vi "BATTERY EMULATOR AUTO MODE.vi"(8 "error IN":errorcluster) -> (0 "error out":errorcluster)   [LabVIEW 2018]
uses:
  Controls/MODEL CONTROL.ctl
  3e16ebac-11a9-43af-ac05-86c9ef550ade.vi
  17a302df-ff61-441d-8d7b-7ff2f5324251.vi
  a2baa657-6743-459a-891e-8081dcc02569.vi
  93341af7-0d01-4cec-89d3-509ad52480dd.vi
  <vilib>/xnet/xnet.llb/XNET Create Session (Signal Input Single-point).vi
  <vilib>/xnet/xnet.llb/XNET Read (Signal Single-point).vi
  <vilib>/xnet/xnet.llb/XNET Create Session (Signal Output Single-point).vi
  <vilib>/xnet/xnet.llb/XNET Write (Signal Single-point).vi
panel:
  in  "UPLOAD DATA":bool
  out "MESSAGES":string
  out "CP POWER":string
  out "CP CURRENT":string
  out "CP VOLTAGE":string
  out "CI POWER":string
  out "CI CURRENT":string
  out "CI VOLTAGE":string
  out "CV POWER":string
  out "CV CURRENT":string
  out "CV VOLTAGE":string
  out "CONTROL SELECTION":string
  out "HVHC SELECTION":string
  in  "CP POWER":string
  in  "CP CURRENT":string
  in  "CP VOLTAGE":string
  in  "CI POWER":string
  in  "CI CURRENT":string
  in  "CI VOLTAGE":string
  in  "CV POWER":string
  in  "CV CURRENT":string
  in  "CV VOLTAGE":string
  in  "CONTROL SELECTION":string(combo)
  in  "HVHC SELECTION":string(combo)
  out "Headline":string
  in  "Save Button":bool
  in  "MODEL SELECTION":string(combo)
  # "BATTERY EMULATOR CONTROLS"
  # "BATTERY EMULATOR DATA"
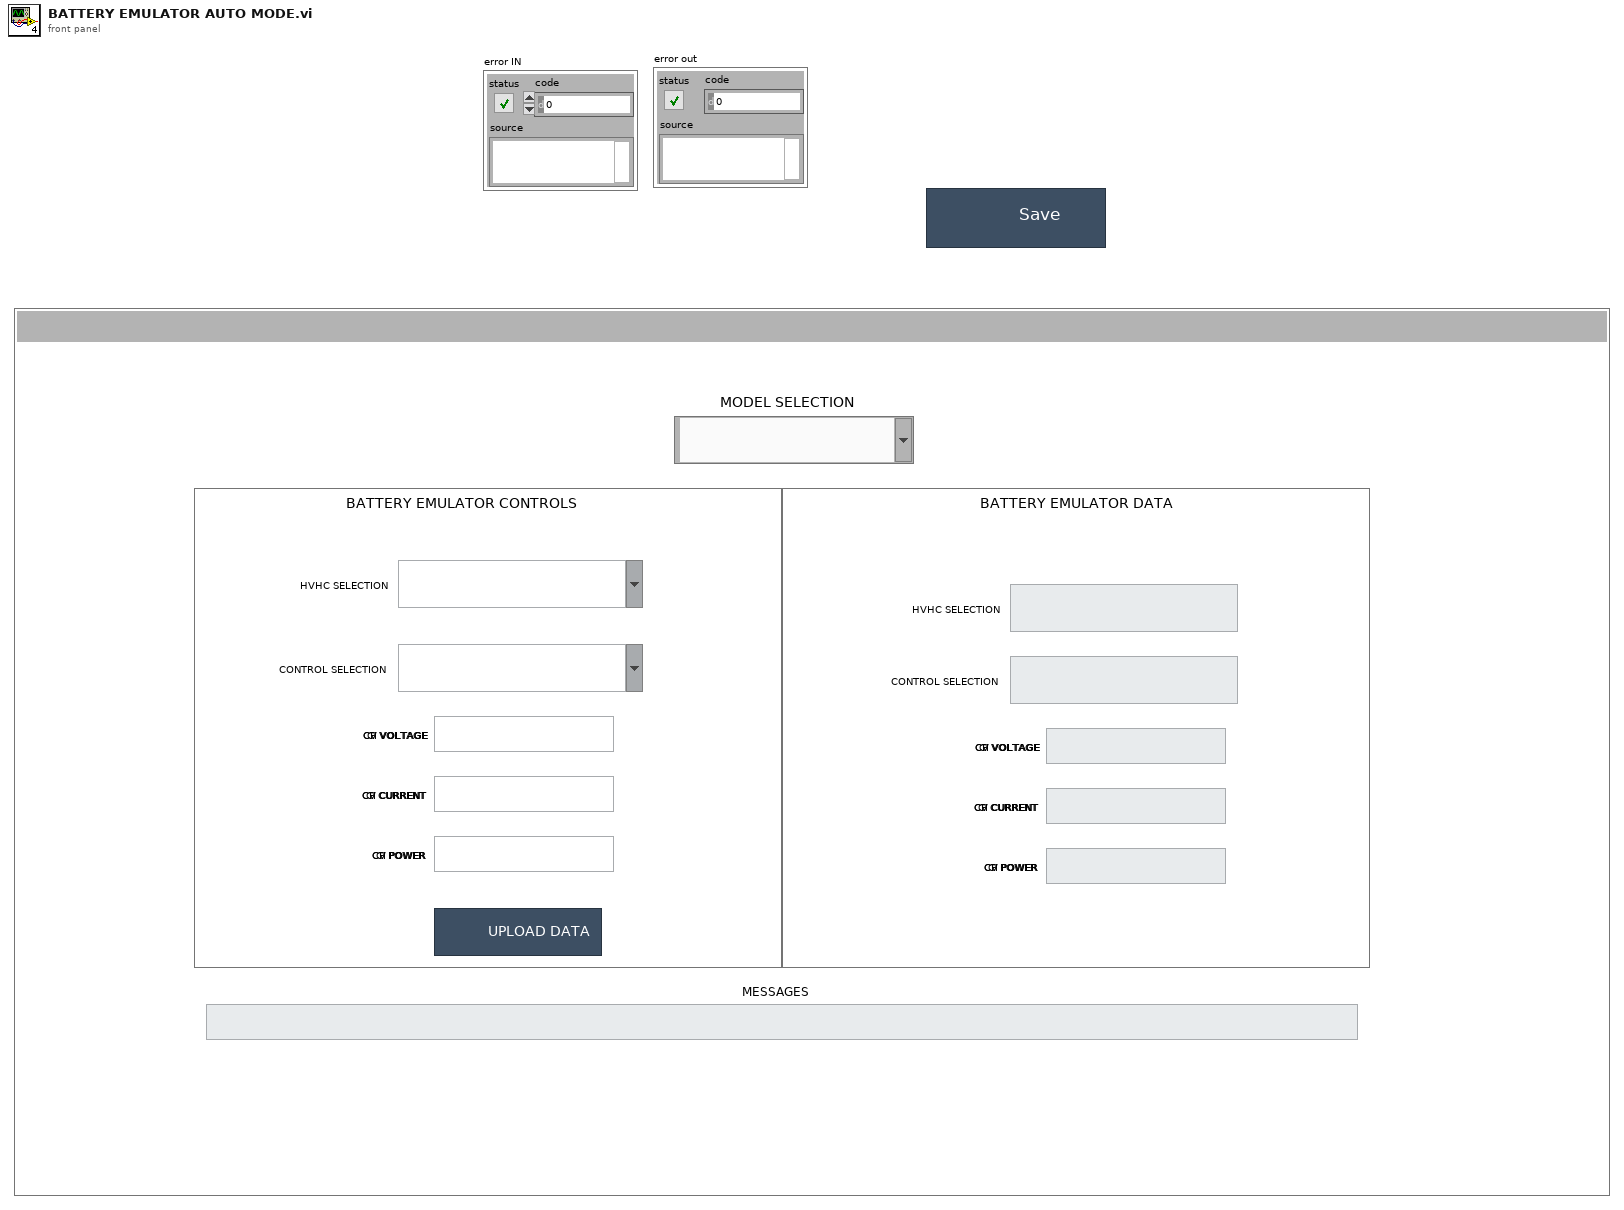
[diagram p1: front panel]
types:
  T1 = enum32{"Invalid", "Standard", "Closed", "Hidden", "Minimized", "Maximized"}
  T2 = enum32{"invalid app kind", "Development System", "Run Time System", "Student Edition", "Embedded LabVIEW", "Evaluation", "Custom"}
  T3 = typedef "MODEL CONTROL.ctl" = enum16{"OPEN", "READ", "WRITE", "CLOSE"}
  T4 = cluster{"Core":cluster{"Current VI Reference":refnum<vi>, "Close Panel on Exit?":bool}, "CHANGE REQ?":bool, "Your string data":string, "BATTERY EMULATOR":cluster{"HVHC SELECT":string, "CONTROL SELECTION":string, "CV VOLTAGE":string, "CV CURRENT":string, "CV POWER":string, "CI VOLTAGE":string, "CI CURRENT":string, "CI POWER":string, "CP VOLTAGE":string, "CP CURRENT":string, "CP POWER":string}, "File paths":cluster{"Base file path":path, "Model File path":path}, "DATA WRITE COUNT":i32, "MESSAGES":string}
  T5 = cluster{"HVHC SELECT":string, "CONTROL SELECTION":string, "CV VOLTAGE":string, "CV CURRENT":string, "CV POWER":string, "CI VOLTAGE":string, "CI CURRENT":string, "CI POWER":string, "CP VOLTAGE":string, "CP CURRENT":string, "CP POWER":string}
  T6 = cluster{"Base file path":path, "Model File path":path}
  T7 = cluster{"Current VI Reference":refnum<vi>, "Close Panel on Exit?":bool}
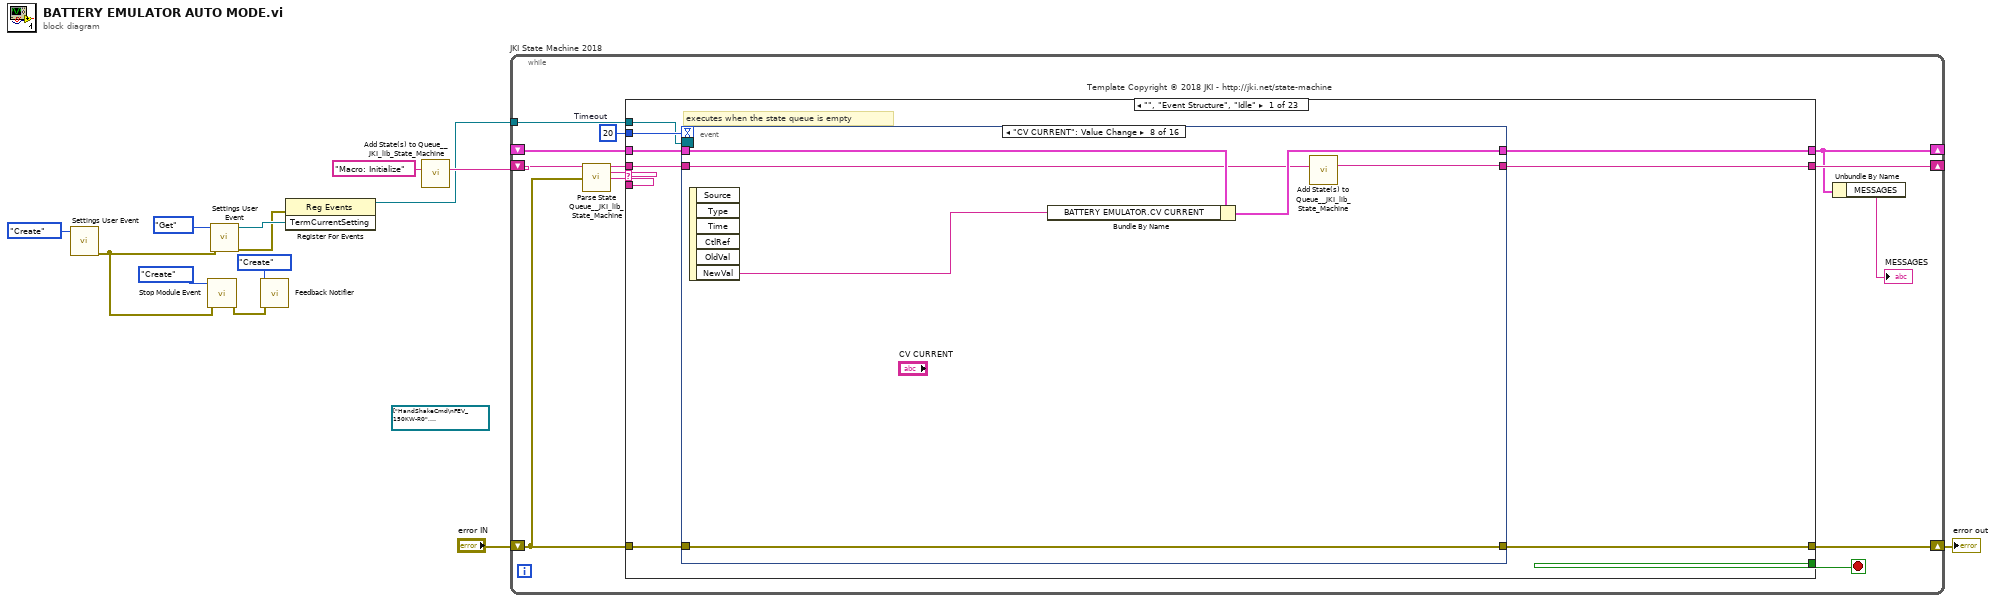
[diagram p0: block diagram]
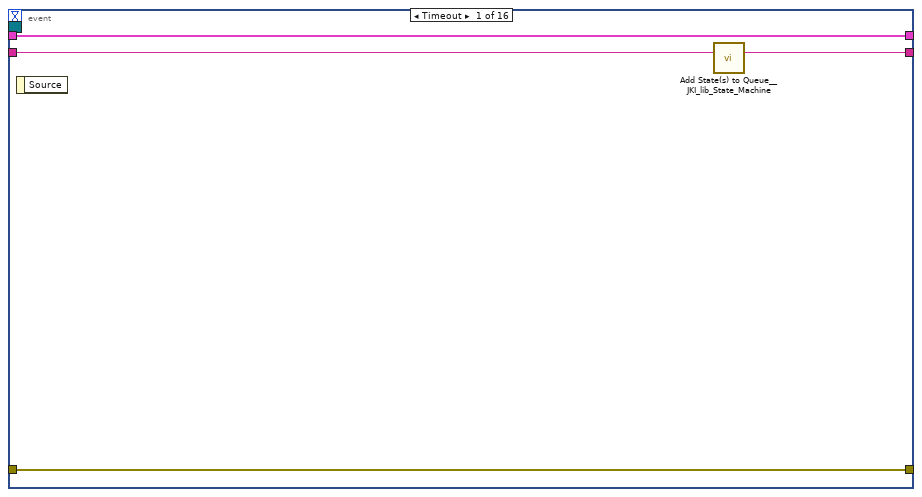
[diagram p2: hidden frame]
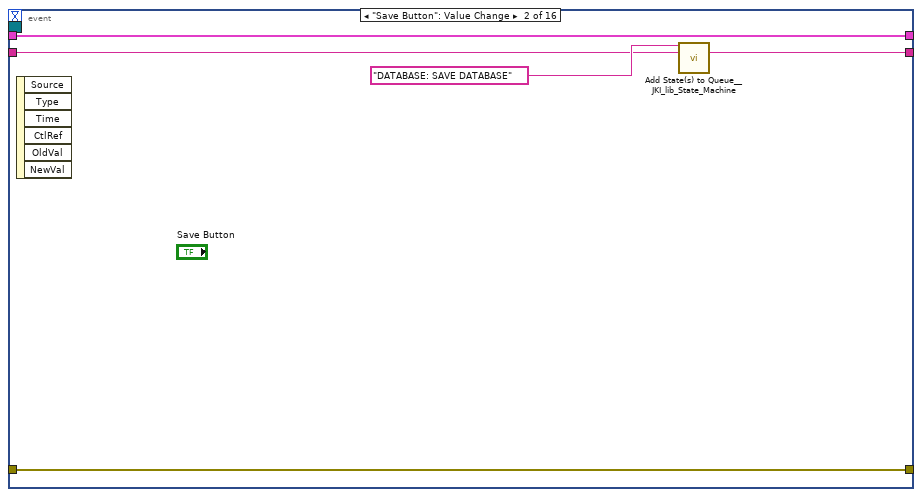
[diagram p3: hidden frame]
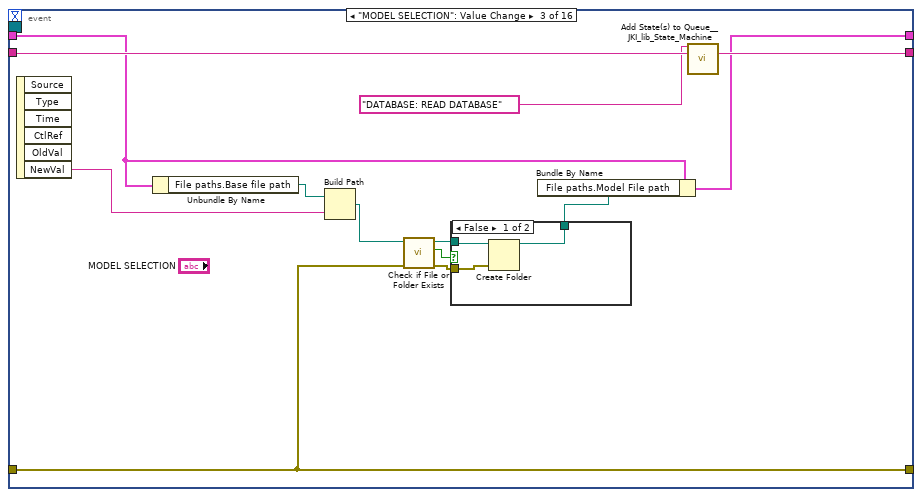
[diagram p4: hidden frame]
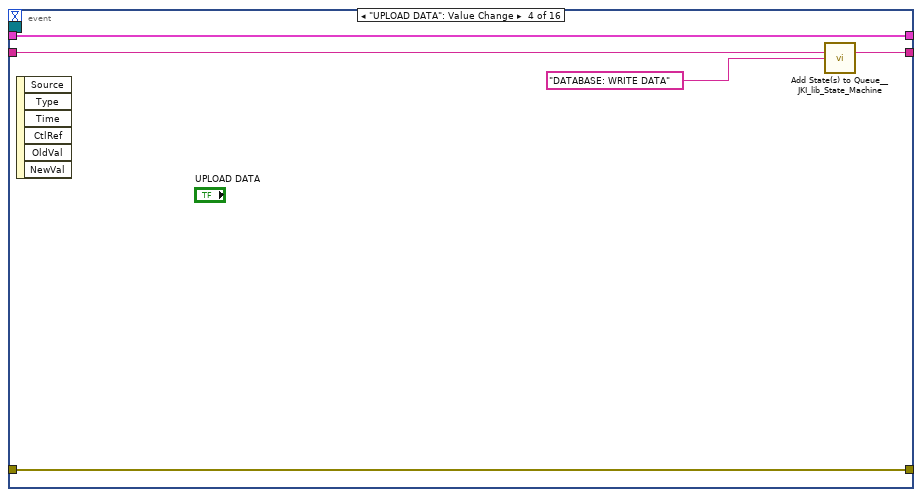
[diagram p6: hidden frame]
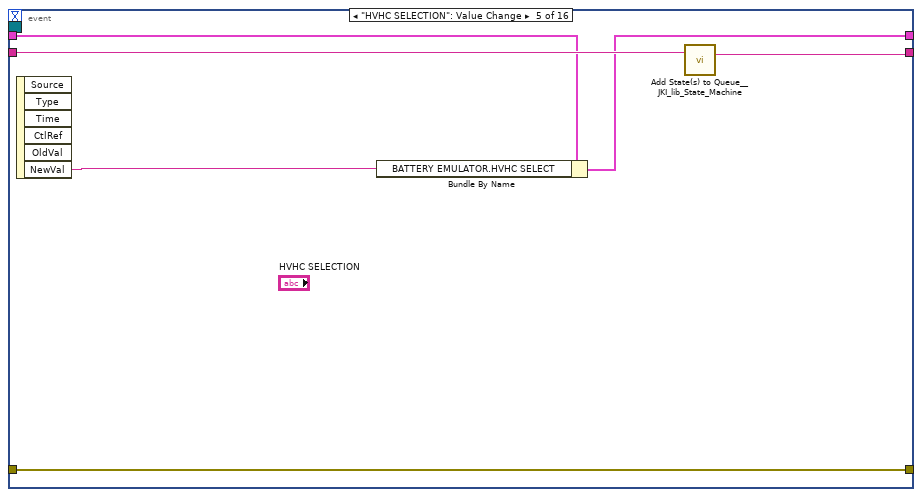
[diagram p7: hidden frame]
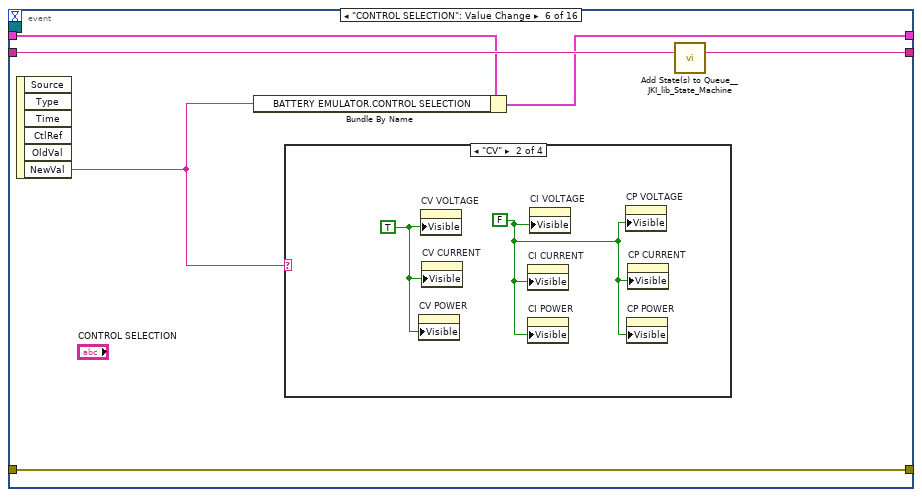
[diagram p8: hidden frame]
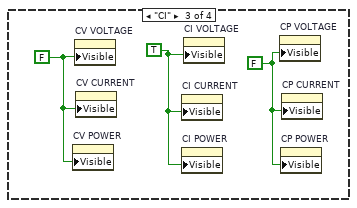
[diagram p10: hidden frame]
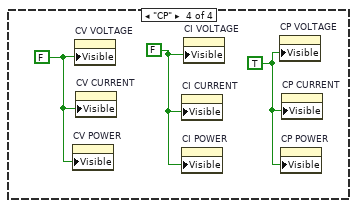
[diagram p11: hidden frame]
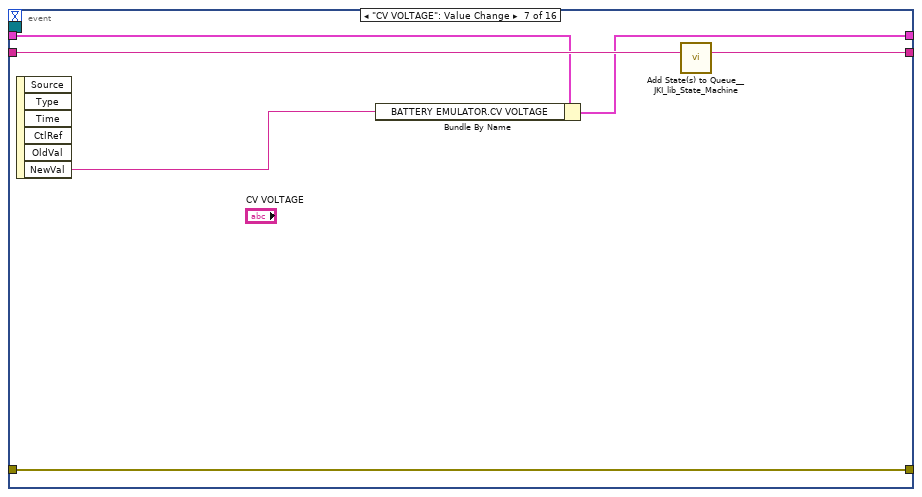
[diagram p12: hidden frame]
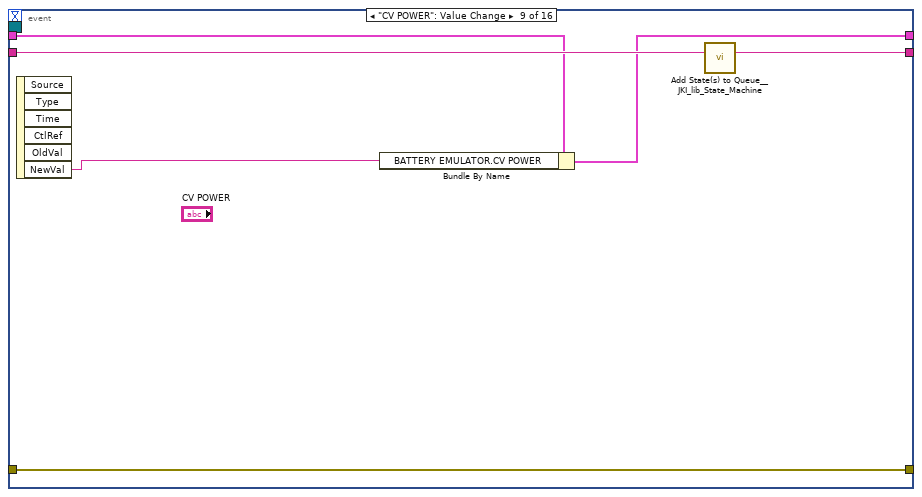
[diagram p13: hidden frame]
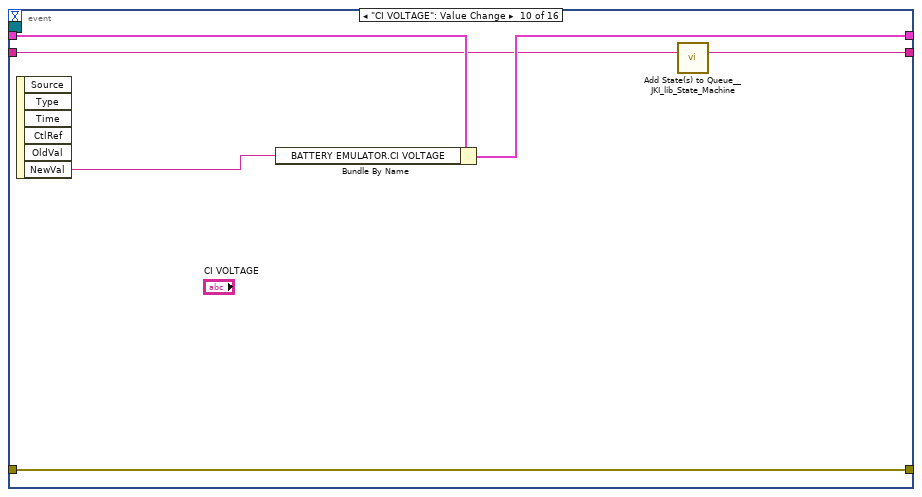
[diagram p14: hidden frame]
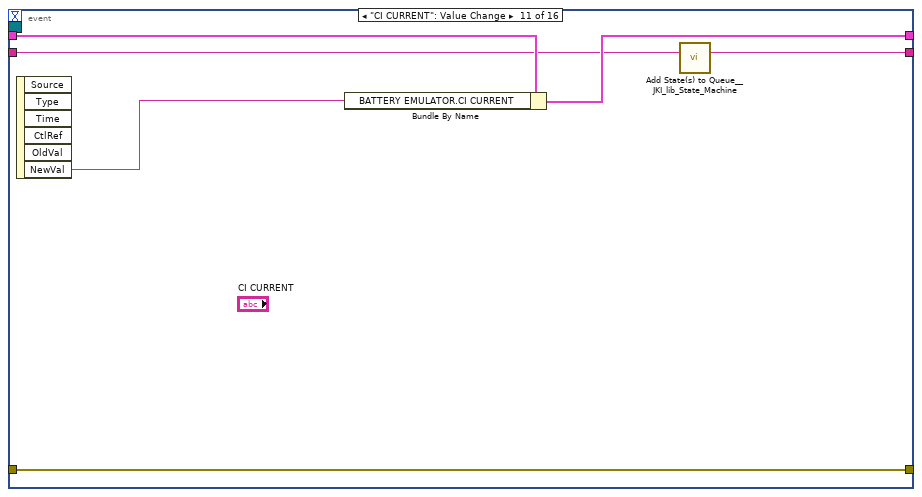
[diagram p15: hidden frame]
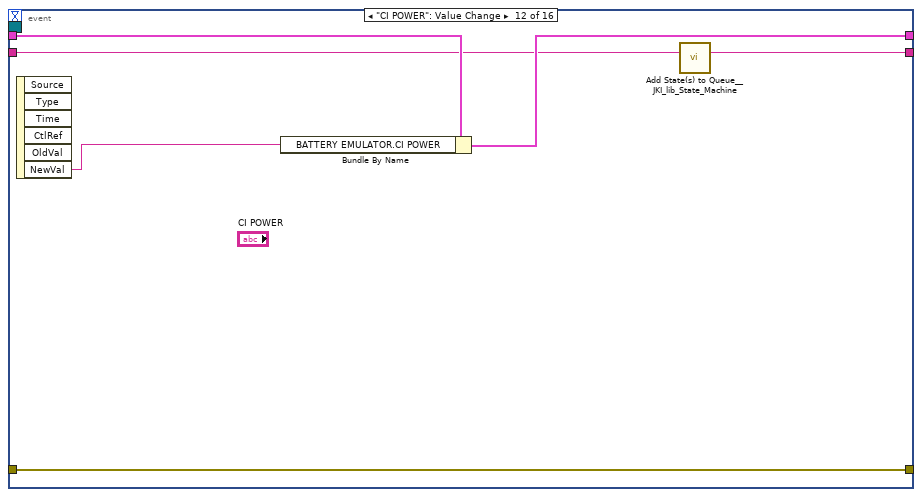
[diagram p16: hidden frame]
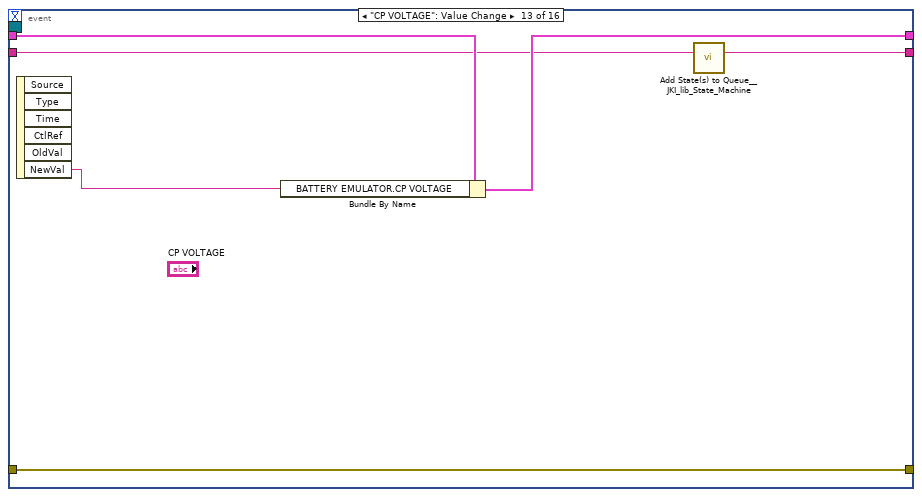
[diagram p17: hidden frame]
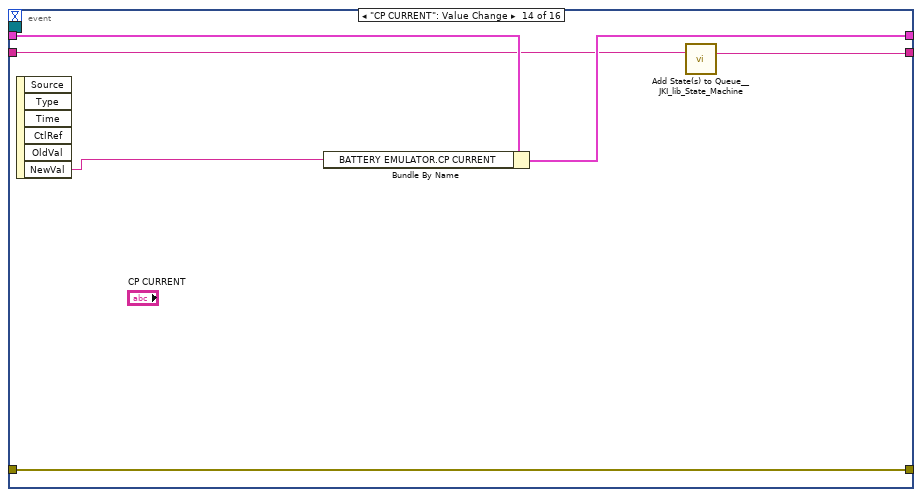
[diagram p18: hidden frame]
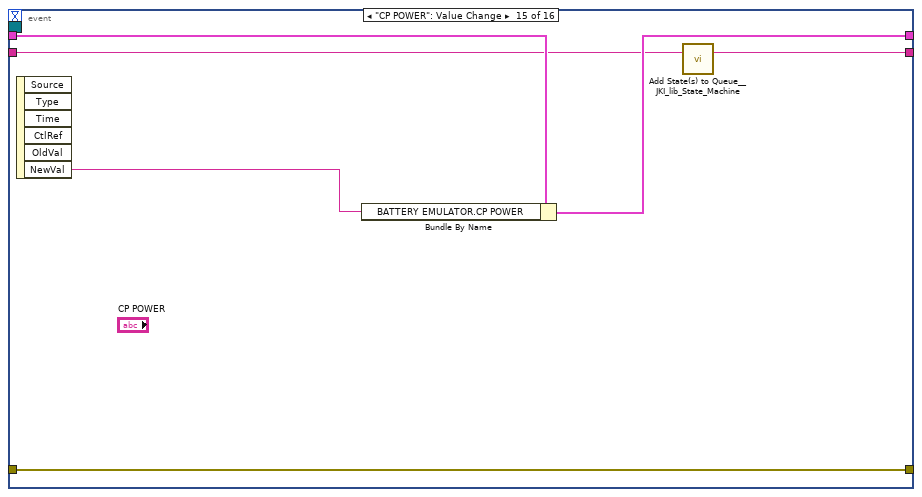
[diagram p19: hidden frame]
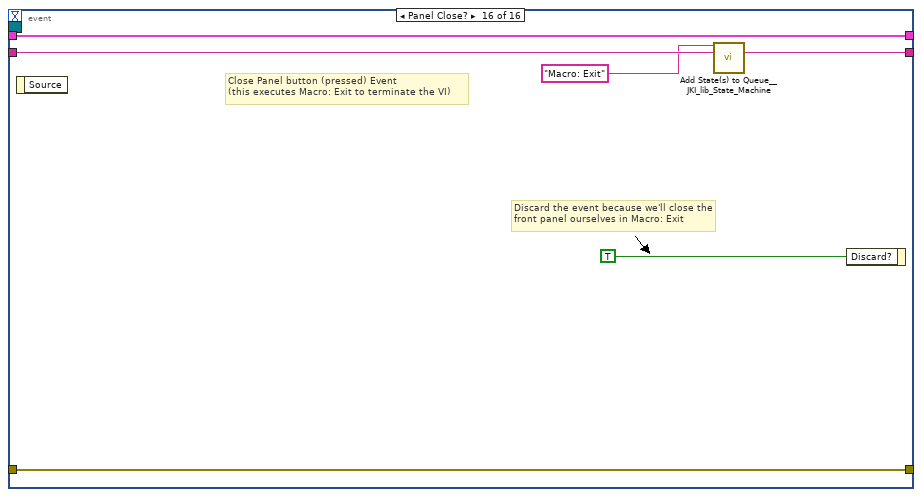
[diagram p20: hidden frame]
diagram:
  (unwired) refnum<k21>[] ["HandShakeCmd\nFEV_150KW-R0", "RemoteDisplaySel\nFEV_150KW-R0", "Select_HVHC", "Select_CVCICP", "CV_SetCurrentLimit\nFEV_150KW-R0", "CV_SetPowerLimit\nFEV_150KW-R0", "CV_SetVoltage\nFEV_150KW-R0", "B_RemoteToDcps.Reserved\nFEV_150KW-R0", "CI_SetCurrent\nFEV_150KW-R0", "CI_SetPowerLimit\nFEV_150KW-R0", "CI_SetVoltageLimit\nFEV_150KW-R0", "C_RemoteToDcps.Reserved\nFEV_150KW-R0", "CP_SetCurrentLimit\nFEV_150KW-R0", "CP_SetPower\nFEV_150KW-R0", "CP_SetVoltageLimit\nFEV_150KW-R0", "D_RemoteToDcps.UpdateCmd\nFEV_150KW-R0", "HandShakeAcknowledge\nFEV_150KW-R0", "RemoteDisplaySelAck\nFEV_150KW-R0", "Select_CVCICPAck\nFEV_150KW-R0", "Select_HVHC_Ack\nFEV_150KW-R0", "CV_SetCurrentLimitAck\nFEV_150KW-R0", "CV_SetPowerLimitAck\nFEV_150KW-R0", "CV_SetVoltageAck\nFEV_150KW-R0", "PowerSwitchONStatus\nFEV_150KW-R0", "CI_SetCurrentAck\nFEV_150KW-R0", "CI_SetPowerLimitAck\nFEV_150KW-R0", "CI_SetVoltageLimitAck\nFEV_150KW-R0", "ErrorControlSelErr\nFEV_150KW-R0", "ErrorCurSetOutofRange\nFEV_150KW-R0", "ErrorNotInRemoteMode\nFEV_150KW-R0", "ErrorPowerSetOutofRange\nFEV_150KW-R0", "ErrorVoltSetOutofRange\nFEV_150KW-R0", "ErrorWrongHVSel\nFEV_150KW-R0", "Reserved_Status\nFEV_150KW-R0", "CP_SetCurrentLimitAck\nFEV_150KW-R0", "CP_SetPowerAck\nFEV_150KW-R0", "CP_SetVoltageLimitAck\nFEV_150KW-R0", "UpdateCmdAcknowledge\nFEV_150KW-R0", "OutputCurrent\nFEV_150KW-R0", "OutputPower\nFEV_150KW-R0", "OutputVoltage\nFEV_150KW-R0", "StatusDcpsFault\nFEV_150KW-R0", "StatusDcpsON\nFEV_150KW-R0", "StatusDcpsOverload\nFEV_150KW-R0", "StatusDcpsTrip\nFEV_150KW-R0", "StatusHCHV_selection\nFEV_150KW-R0", "StatusInputOverVolt\nFEV_150KW-R0", "StatusInputUnderVolt\nFEV_150KW-R0", "StatusMainsHealthy\nFEV_150KW-R0", "StatusOutputOverVolt\nFEV_150KW-R0", "StatusOutputUnderVolt\nFEV_150KW-R0", "StatusOverTemperature\nFEV_150KW-R0", "StatusRemoteLocal\nFEV_150KW-R0"] ("Sigs 3")
  n1 = call "Settings User Event.vi"("Action"=enum16{"Create", "Get", "Destroy"}."Create") -> ("error out"=w6:errorcluster)  [unwired: 9 in, 1 out]
  n2 = call "Stop Module Event.vi"("error in (no error)"=w6, "Action"=enum16{"Create", "Get", "Destroy"}."Create") -> ("error out"=w5:errorcluster)  [unwired: 8 in, 1 out]
  n3 = call "Settings User Event.vi"("error in (no error)"=w6, "Action"=enum16{"Create", "Get", "Destroy"}."Get") -> ("error out"=w8:errorcluster, "TermCurrentSetting"=w9:refnum<user-event>)  [unwired: 8 in]
  n4 = call "Feedback Notifier.vi"("error in (no error)"=w5, "Action"=enum16{"Create", "Get", "Destroy"}."Create") -> ()  [unwired: 8 in, 2 out]
  n5 = register-events(error in=w8, w9) -> (reference out=w3:refnum<event-registration>)  [unwired: 1 in, 1 out]
  n6 = call <vilib>:"Add State(s) to Queue__JKI_lib_State_Machine.vi"("State(s) in (\"\")"="Macro: Initialize") -> ("States Out"=w13:string)  [unwired: 14 in]
  n7 = while "JKI State Machine 2018" {
    shift-right: [w15] -> _
    shift-left: _ -> [w19]
    shift-right: [w22] -> w1
    shift-left: "error IN" -> [w17]
    shift-right: [w21] -> _
    shift-left: w13 -> [w23]
    tunnel: w3 -> [w16]
    stop <- w20 stop-if-true
    w18 = 20  # Timeout
    # "Template Copyright © 2018 JKI - http://jki.net/state-machine"
    n8 = call <vilib>:"Parse State Queue__JKI_lib_State_Machine.vi"("State Queue"=w23, "Error In (no error)"=w17) -> ("Remaining States"=w25:string, "Current State"=w26:string, "Arguments"=w24:string)  [unwired: 11 in]
    n9 = case shown="\"\", \"Event Structure\", \"Idle\"" w26 {
      selector: w26 -> [_ _ w150 _ _ _ _ _ _ _ _ _ _ _ _ _ _ _ _ _ _ _ _]
      tunnel: w25 -> [w34 w149 w154 w173 w179 w184 w188 w199 w205 w209 w213 w219 w223 w226 w249 w261 w330 w335 w352 w366 w391 w438 w506]
      tunnel: w24 -> [_ _ _ _ _ _ _ _ _ _ _ _ _ _ w244 w255 _ _ _ _ _ _ _]
      tunnel: w19 -> [w32 w146 w152 w166 w176 w182 w185 _ w200 w206 w211 w217 w220 w238 w247 w257 w327 w332 w340 w363 w370 w402 w476]
      tunnel: [w31 w147 w156 w170 errorcluster {"status"=FALSE, "code"=0, "source"=""} ("error out") w181 w186 w196 w201 w207 w210 w214 w221 w239 w245 w258 w328 w333 w344 w364 w385 w428 w477] -> w22
      tunnel: w17 -> [w30 w147 w155 w170 w175 w181 w186 w196 w202 w207 w210 w215 w221 w236 w246 w259 w328 w333 w345 w364 w389 w410 w478]
      tunnel: [w33 w148 w153 w172 w178 w183 w187 w198 w204 w208 w212 w218 w222 w243 w248 w260 w329 w334 w351 w365 w390 w437 w505] -> w21
      tunnel: [_ _ _ _ _ TRUE _ _ _ _ _ _ _ _ _ _ _ _ _ _ _ _ _] -> w20
      tunnel: [w29 w146 w152 w171 w176 w182 w185 w197 w200 w206 w211 w217 w220 w237 w247 w257 w327 w332 w339 w363 w369 w401 w476] -> w15
      tunnel: w18 -> [w28 _ _ _ _ _ _ _ _ _ _ _ _ _ _ _ _ _ _ _ _ _ _]
      tunnel: w16 -> [w27 _ _ _ _ _ _ _ _ _ _ w216 _ _ _ _ _ _ _ _ _ _ _]
      frame "", "Event Structure", "Idle" {
        # "executes when the state queue is empty"
        n10 = event shown="[7] \"CV CURRENT\": Value Change" {
          selector: w27 -> [_ _ _ _ _ _ _ _ _ _ _ _ _ _ _ _]
          dyn-events: _ -> [_ _ _ _ _ _ _ _ _ _ _ _ _ _ _ _]
          timeout: w28 -> [_ _ _ _ _ _ _ _ _ _ _ _ _ _ _ _]
          tunnel: w34 -> [w38 w40 w55 w63 w70 w75 w90 w93 w101 w105 w111 w116 w122 w128 w134 w145]
          tunnel: [w37 w41 w56 w64 w71 w76 w91 w94 w102 w106 w112 w117 w123 w129 w135 w144] -> w33
          tunnel: w32 -> [w35 w42 w51 w65 w69 w74 w89 w97 w100 w109 w114 w120 w126 w132 w138 w142]
          tunnel: [w36 w39 w48 w62 w66 w77 w86 w92 w103 w104 w115 w121 w127 w133 w139 w143] -> w31
          tunnel: w30 -> [w36 w39 w48 w62 w66 w77 w86 w92 w103 w104 w115 w121 w127 w133 w139 w143]
          tunnel: [w35 w42 w50 w65 w67 w73 w87 w96 w99 w108 w113 w118 w125 w131 w137 w142] -> w29
          event Timeout {
            n11 = event-data() -> ()  [unwired: 1 in, 1 out]
            n12 = call <vilib>:"Add State(s) to Queue__JKI_lib_State_Machine.vi"("State(s) in (\"\")"=w38) -> ("States Out"=w37:string)  [unwired: 14 in]
          }
          event "Save Button": Value Change {
            n13 = event-data() -> ()  [unwired: 1 in, 6 out]
            n14 = call <vilib>:"Add State(s) to Queue__JKI_lib_State_Machine.vi"("State(s) in Front (\"\")"="DATABASE: SAVE DATABASE", "State(s) in (\"\")"=w40) -> ("States Out"=w41:string)  [unwired: 13 in]
          }
          event "MODEL SELECTION": Value Change {
            n15 = event-data() -> ("NewVal"=w52:string)  [unwired: 1 in, 5 out]
            n16 = Unbundle By Name(w51) -> ("File paths.Base file path"=w53:path)
            n17 = Build Path(base path=w53, name or relative path=w52) -> (appended path=w49:path)
            n18 = call <vilib>:"Check if File or Folder Exists.vi"("error in (no error)"=w48, "path"=w49) -> ("error out"=w46:errorcluster, "file or folder exists?"=w45:bool, "dup path"=w47:path)  [unwired: 7 in]
            n19 = case shown="False" w45 {
              tunnel: w47 -> [w58 w60]
              tunnel: w46 -> [w59 _]
              tunnel: [w57 w60] -> w44
              frame False {
                n20 = Create Folder(path (use dialog)=w58, error in=w59) -> (created path=w57:path)  [unwired: 1 in, 2 out]
              }
              frame True {
              }
            }
            n21 = Bundle By Name(cluster=w51, "File paths.Model File path"=w44) -> (w50:T4)
            n22 = call <vilib>:"Add State(s) to Queue__JKI_lib_State_Machine.vi"("State(s) in Front (\"\")"="DATABASE: READ DATABASE", "State(s) in (\"\")"=w55) -> ("States Out"=w56:string)  [unwired: 13 in]
          }
          event "UPLOAD DATA": Value Change {
            n23 = event-data() -> ()  [unwired: 1 in, 6 out]
            n24 = call <vilib>:"Add State(s) to Queue__JKI_lib_State_Machine.vi"("State(s) in (\"\")"=w63, "State(s) at Back (\"\")"="DATABASE: WRITE DATA") -> ("States Out"=w64:string)  [unwired: 13 in]
          }
          event "HVHC SELECTION": Value Change {
            n25 = event-data() -> ("NewVal"=w68:string)  [unwired: 1 in, 5 out]
            n26 = Bundle By Name(cluster=w69, "BATTERY EMULATOR.HVHC SELECT"=w68) -> (w67:T4)
            n27 = call <vilib>:"Add State(s) to Queue__JKI_lib_State_Machine.vi"("State(s) in (\"\")"=w70) -> ("States Out"=w71:string)  [unwired: 14 in]
          }
          event "CONTROL SELECTION": Value Change {
            n28 = event-data() -> ("NewVal"=w72:string)  [unwired: 1 in, 5 out]
            n29 = Bundle By Name(cluster=w74, "BATTERY EMULATOR.CONTROL SELECTION"=w72) -> (w73:T4)
            n30 = case shown="\"CV\"" w72 {
              frame "False", Default {
              }
              frame "CV" {
                w78 = FALSE ("Visible")
                w79 = TRUE ("Visible")
                n31 = property on="CV POWER" class="Str"("Visible"=w79) -> ()  [unwired: 2 in, 2 out]
                n32 = property on="CV VOLTAGE" class="Str"("Visible"=w79) -> ()  [unwired: 2 in, 2 out]
                n33 = property on="CV CURRENT" class="Str"("Visible"=w79) -> ()  [unwired: 2 in, 2 out]
                n34 = property on="CI CURRENT" class="Str"("Visible"=w78) -> ()  [unwired: 2 in, 2 out]
                n35 = property on="CI POWER" class="Str"("Visible"=w78) -> ()  [unwired: 2 in, 2 out]
                n36 = property on="CI VOLTAGE" class="Str"("Visible"=w78) -> ()  [unwired: 2 in, 2 out]
                n37 = property on="CP VOLTAGE" class="Str"("Visible"=w78) -> ()  [unwired: 2 in, 2 out]
                n38 = property on="CP POWER" class="Str"("Visible"=w78) -> ()  [unwired: 2 in, 2 out]
                n39 = property on="CP CURRENT" class="Str"("Visible"=w78) -> ()  [unwired: 2 in, 2 out]
              }
              frame "CI" {
                w80 = FALSE ("Visible")
                w81 = TRUE ("Visible")
                w82 = FALSE ("Visible")
                n40 = property on="CV POWER" class="Str"("Visible"=w82) -> ()  [unwired: 2 in, 2 out]
                n41 = property on="CV VOLTAGE" class="Str"("Visible"=w82) -> ()  [unwired: 2 in, 2 out]
                n42 = property on="CV CURRENT" class="Str"("Visible"=w82) -> ()  [unwired: 2 in, 2 out]
                n43 = property on="CI CURRENT" class="Str"("Visible"=w81) -> ()  [unwired: 2 in, 2 out]
                n44 = property on="CI POWER" class="Str"("Visible"=w81) -> ()  [unwired: 2 in, 2 out]
                n45 = property on="CI VOLTAGE" class="Str"("Visible"=w81) -> ()  [unwired: 2 in, 2 out]
                n46 = property on="CP VOLTAGE" class="Str"("Visible"=w80) -> ()  [unwired: 2 in, 2 out]
                n47 = property on="CP POWER" class="Str"("Visible"=w80) -> ()  [unwired: 2 in, 2 out]
                n48 = property on="CP CURRENT" class="Str"("Visible"=w80) -> ()  [unwired: 2 in, 2 out]
              }
              frame "CP" {
                w83 = TRUE ("Visible")
                w84 = FALSE ("Visible")
                w85 = FALSE ("Visible")
                n49 = property on="CV POWER" class="Str"("Visible"=w85) -> ()  [unwired: 2 in, 2 out]
                n50 = property on="CV VOLTAGE" class="Str"("Visible"=w85) -> ()  [unwired: 2 in, 2 out]
                n51 = property on="CV CURRENT" class="Str"("Visible"=w85) -> ()  [unwired: 2 in, 2 out]
                n52 = property on="CI CURRENT" class="Str"("Visible"=w84) -> ()  [unwired: 2 in, 2 out]
                n53 = property on="CI POWER" class="Str"("Visible"=w84) -> ()  [unwired: 2 in, 2 out]
                n54 = property on="CI VOLTAGE" class="Str"("Visible"=w84) -> ()  [unwired: 2 in, 2 out]
                n55 = property on="CP VOLTAGE" class="Str"("Visible"=w83) -> ()  [unwired: 2 in, 2 out]
                n56 = property on="CP POWER" class="Str"("Visible"=w83) -> ()  [unwired: 2 in, 2 out]
                n57 = property on="CP CURRENT" class="Str"("Visible"=w83) -> ()  [unwired: 2 in, 2 out]
              }
            }
            n58 = call <vilib>:"Add State(s) to Queue__JKI_lib_State_Machine.vi"("State(s) in (\"\")"=w75) -> ("States Out"=w76:string)  [unwired: 14 in]
          }
          event "CV VOLTAGE": Value Change {
            n59 = event-data() -> ("NewVal"=w88:string)  [unwired: 1 in, 5 out]
            n60 = Bundle By Name(cluster=w89, "BATTERY EMULATOR.CV VOLTAGE"=w88) -> (w87:T4)
            n61 = call <vilib>:"Add State(s) to Queue__JKI_lib_State_Machine.vi"("State(s) in (\"\")"=w90) -> ("States Out"=w91:string)  [unwired: 14 in]
          }
          event "CV CURRENT": Value Change {
            n62 = event-data() -> ("NewVal"=w95:string)  [unwired: 1 in, 5 out]
            n63 = Bundle By Name(cluster=w97, "BATTERY EMULATOR.CV CURRENT"=w95) -> (w96:T4)
            n64 = call <vilib>:"Add State(s) to Queue__JKI_lib_State_Machine.vi"("State(s) in (\"\")"=w93) -> ("States Out"=w94:string)  [unwired: 14 in]
          }
          event "CV POWER": Value Change {
            n65 = event-data() -> ("NewVal"=w98:string)  [unwired: 1 in, 5 out]
            n66 = Bundle By Name(cluster=w100, "BATTERY EMULATOR.CV POWER"=w98) -> (w99:T4)
            n67 = call <vilib>:"Add State(s) to Queue__JKI_lib_State_Machine.vi"("State(s) in (\"\")"=w101) -> ("States Out"=w102:string)  [unwired: 14 in]
          }
          event "CI VOLTAGE": Value Change {
            n68 = event-data() -> ("NewVal"=w107:string)  [unwired: 1 in, 5 out]
            n69 = Bundle By Name(cluster=w109, "BATTERY EMULATOR.CI VOLTAGE"=w107) -> (w108:T4)
            n70 = call <vilib>:"Add State(s) to Queue__JKI_lib_State_Machine.vi"("State(s) in (\"\")"=w105) -> ("States Out"=w106:string)  [unwired: 14 in]
          }
          event "CI CURRENT": Value Change {
            n71 = event-data() -> ("NewVal"=w110:string)  [unwired: 1 in, 5 out]
            n72 = Bundle By Name(cluster=w114, "BATTERY EMULATOR.CI CURRENT"=w110) -> (w113:T4)
            n73 = call <vilib>:"Add State(s) to Queue__JKI_lib_State_Machine.vi"("State(s) in (\"\")"=w111) -> ("States Out"=w112:string)  [unwired: 14 in]
          }
          event "CI POWER": Value Change {
            n74 = event-data() -> ("NewVal"=w119:string)  [unwired: 1 in, 5 out]
            n75 = Bundle By Name(cluster=w120, "BATTERY EMULATOR.CI POWER"=w119) -> (w118:T4)
            n76 = call <vilib>:"Add State(s) to Queue__JKI_lib_State_Machine.vi"("State(s) in (\"\")"=w116) -> ("States Out"=w117:string)  [unwired: 14 in]
          }
          event "CP VOLTAGE": Value Change {
            n77 = event-data() -> ("NewVal"=w124:string)  [unwired: 1 in, 5 out]
            n78 = Bundle By Name(cluster=w126, "BATTERY EMULATOR.CP VOLTAGE"=w124) -> (w125:T4)
            n79 = call <vilib>:"Add State(s) to Queue__JKI_lib_State_Machine.vi"("State(s) in (\"\")"=w122) -> ("States Out"=w123:string)  [unwired: 14 in]
          }
          event "CP CURRENT": Value Change {
            n80 = event-data() -> ("NewVal"=w130:string)  [unwired: 1 in, 5 out]
            n81 = Bundle By Name(cluster=w132, "BATTERY EMULATOR.CP CURRENT"=w130) -> (w131:T4)
            n82 = call <vilib>:"Add State(s) to Queue__JKI_lib_State_Machine.vi"("State(s) in (\"\")"=w128) -> ("States Out"=w129:string)  [unwired: 14 in]
          }
          event "CP POWER": Value Change {
            n83 = event-data() -> ("NewVal"=w136:string)  [unwired: 1 in, 5 out]
            n84 = Bundle By Name(cluster=w138, "BATTERY EMULATOR.CP POWER"=w136) -> (w137:T4)
            n85 = call <vilib>:"Add State(s) to Queue__JKI_lib_State_Machine.vi"("State(s) in (\"\")"=w134) -> ("States Out"=w135:string)  [unwired: 14 in]
          }
          event Panel Close? {
            # "Discard the event because we'll close the front panel ourselves in Macro: Exit"
            # "Close Panel button (pressed) Event\n(this executes Macro: Exit to terminate the VI)"
            n86 = event-data() -> ()  [unwired: 1 in, 1 out]
            n87 = call <vilib>:"Add State(s) to Queue__JKI_lib_State_Machine.vi"("State(s) in Front (\"\")"="Macro: Exit", "State(s) in (\"\")"=w145) -> ("States Out"=w144:string)  [unwired: 13 in]
            n88 = event-data("Discard?"=TRUE) -> ()  [unwired: 1 in, 1 out]
          }
        }
      }
      frame "---------- Core ----------" {
        # "Do not put any code in this frame.\n(it is a separator no-op)"
        n89 = call <vilib>:"Add State(s) to Queue__JKI_lib_State_Machine.vi"("State(s) in (\"\")"=w149) -> ("States Out"=w148:string)  [unwired: 14 in]
      }
      frame Default {
        w159 = 42 items=["No error", "Argument error", "Memory is full", "Out of zone", "End of file", "File already open", "Generic file I/O error", "File not found", "File permission error", "Disk is full", "Duplicate path", "Too many files open", "System feature not enabled", "Resource file not found", "Cannot add resource", "Resource not found", "Image not found", "Image memory error", "Pen does not exist", "Config type invalid", "Config token not found", "Config parse error", "Config memory error", "Bad external code format", "Bad external code offset", "External code not present", "Null window", "Destroy window error", "Null menu", "Print aborted", "Bad print record", "Print driver error", "Windows error during printing", "Memory error during printing", "Print dialog error", "Generic print error", "Invalid device refnum", "Device not found", "Device parameter error", "Device unit error", "Cannot open device", "Device call aborted", "Generic error", "Cancelled by user", "Object ID too low", "Object ID too high", "Object not in heap", "Unknown heap", "Unknown object (invalid DefProc)", "Unknown object (DefProc not in table)", "Message out of range", "Invalid (null) method", "Unknown message", "Manager call not supported", "Bad address", "Network operation in progress", "Network operation timed out", "Connection is busy", "Network attribute not supported", "Network error", "Address in use", "System out of memory", "Connection aborted", "Connection refused", "Not connected", "Already connected", "Connection closed", "Initialization error (interapplication manager)", "Bad occurrence", "Wait on unbound occurrence handler", "Occurrence queue overflow", "Datalog type conflict", "Unused", "Unrecognized type (interapplication manager)", "Memory corrupt", "Failed to make temporary DLL", "Old CIN version", "Drag socket not found", "Failed to load drop-object", "Failed to register OLE object", "Failed to release OLE object", "Format specifier type mismatch", "Unknown format specifier", "Too few format specifiers", "Too many format specifiers", "Scan failed", "Newer CIN version", "Error converting to variant", "Runtime menu error", "Password tampered", "Variant attribute not found", "Incompatible variant data type", "Event data is not available", "Event Store is not present", "Occurrence is not found", "Event Queue is not created", "Event info is not available", "Refnum passed is NULL", "Error retrieving Class GUID", "Error retrieving CoClass GUID", "Error retrieving TypeLib GUID.", "Bad built application magic bytes.", "Specific driver is different from the specific driver associated with the Logical Name.", "There is no session opened to the class driver.", "Max Error", "MAX - Error with config objects", "MAX - Error loading configuration", "MAX - Group not supported"]
        # "Current State"
        # "Do not delete, rename, or modify this frame.\n(this is used to capture unhandled states and typos)"
        # "Handle mistyped state name (developer tool)"
        n90 = Format Into String(format string="Software Exception: Unhandled State \"%s\"." ("message"), error in=w155, w150) -> (resulting string=w158:string, error out=w157:errorcluster)  [unwired: 1 in]
        n91 = call <vilib>:"Error Cluster From Error Code.vi"("show call chain? (False)"=TRUE, "error in (no error)"=w157, "error message (\"\")"=w158, "error code (0)"=w159) -> ("error out"=w156:errorcluster)  [unwired: 5 in]
        n92 = call <vilib>:"Add State(s) to Queue__JKI_lib_State_Machine.vi"("State(s) in (\"\")"=w154) -> ("States Out"=w153:string)  [unwired: 14 in]
      }
      frame "Initialize Core Data" {
        # "Do not delete, rename, or modify this frame.\n(this is used to determine panel behavior on exit)"
        # "originally closed?"
        # "exe?"
        # "If panel starts closed or is an EXE, then close it when we exit"
        n93 = property class="VI"() -> ("FP.State"=w163:T1)  [unwired: 2 in, 2 out]
        n94 = property class="App"() -> ("App.Kind"=w169:T2)  [unwired: 2 in, 2 out]
        n95 = control-ref of="Current VI Reference"() -> (w164:refnum<vi>)
        n96 = Equal?(x=w163, y=T1."Closed" ("Front Panel Window:State")) -> (x = y?=w161:bool)
        n97 = Equal?(x=w169, y=T2."Run Time System" ("Application:Kind")) -> (x = y?=w167:bool)
        n98 = Or(x=w161, y=w167) -> (x .or. y?=w165:bool)
        n99 = Bundle By Name(cluster=w166, "Core.Current VI Reference"=w164, "Core.Close Panel on Exit?"=w165) -> (w171:T4)
        n100 = call <vilib>:"Add State(s) to Queue__JKI_lib_State_Machine.vi"("State(s) in (\"\")"=w173) -> ("States Out"=w172:string)  [unwired: 14 in]
      }
      frame "Error Handler" {
        # "Unhandled Error -- Display it"
        # "Handle any errors here.\nYou can also output any states to clean-up after errors occur"
        # "Clear error"
        n101 = call <vilib>:"General Error Handler.vi"("error in (no error)"=w175) -> ()  [unwired: 10 in, 5 out]
        n102 = call <vilib>:"Add State(s) to Queue__JKI_lib_State_Machine.vi"("State(s) in Front (\"\")"="/* Post Error States", "State(s) in (\"\")"=w179) -> ("States Out"=w178:string)  [unwired: 13 in]
      }
      frame "Exit" {
        # "Do not put any code in this frame.\n(No errors that occur here will be handled.)"
        n103 = call <vilib>:"Add State(s) to Queue__JKI_lib_State_Machine.vi"("State(s) in (\"\")"=w184) -> ("States Out"=w183:string)  [unwired: 14 in]
      }
      frame "---------- Data ----------" {
        # "Do not put any code in this frame.\n(It is a separator no-op. You can make a copy of this frame to create a new Data frame)"
        n104 = call <vilib>:"Add State(s) to Queue__JKI_lib_State_Machine.vi"("State(s) in (\"\")"=w188) -> ("States Out"=w187:string)  [unwired: 14 in]
      }
      frame "Data: Initialize" {
        w189 = ""  # MESSAGES
        w190 = 0  # DATA WRITE COUNT
        w191 = T5 {"HVHC SELECT"="", "CONTROL SELECTION"="", "CV VOLTAGE"="", "CV CURRENT"="", "CV POWER"="", "CI VOLTAGE"="", "CI CURRENT"="", "CI POWER"="", "CP VOLTAGE"="", "CP CURRENT"="", "CP POWER"=""}  # BATTERY EMULATOR
        w192 = T6 {"Base file path"=path "", "Model File path"=path ""}  # File paths
        w193 = T7 {"Current VI Reference"=refnum, "Close Panel on Exit?"=FALSE}  # Core
        w195 = TRUE  # CHANGE REQ?
        w194 = ""  # Your string data
        # "do not delete - used by framework"
        # "Data names and types of shift register data are defined by this bundle."
        # "Initialize the shift-register data, here.\n(data names are defined by what you wire into the bundle function)"
        n105 = Bundle("Core"=w193, "CHANGE REQ?"=w195, "Your string data"=w194, "BATTERY EMULATOR"=w191, "File paths"=w192, "DATA WRITE COUNT"=w190, "MESSAGES"=w189) -> (w197:T4)  [unwired: 1 in]
        n106 = call <vilib>:"Add State(s) to Queue__JKI_lib_State_Machine.vi"("State(s) in (\"\")"=w199) -> ("States Out"=w198:string)  [unwired: 14 in]
      }
      frame "Data: Cleanup" {
        # "Cleanup any data and references, here.\n(this is called automatically, by the Macro: Exit)"
        n107 = Unbundle By Name(w200) -> ("Core.Current VI Reference"=w203:refnum<vi>)
        n108 = Close Reference(reference=w203, error in (no error)=w202) -> (error out=w201:errorcluster)
        n109 = call <vilib>:"Add State(s) to Queue__JKI_lib_State_Machine.vi"("State(s) in (\"\")"=w205) -> ("States Out"=w204:string)  [unwired: 14 in]
      }
      frame "---------- Events ----------" {
        # "Do not put any code in this frame.\n(It is a separator no-op. You can make a copy of this frame to create a new UI frame)"
        n110 = call <vilib>:"Add State(s) to Queue__JKI_lib_State_Machine.vi"("State(s) in (\"\")"=w209) -> ("States Out"=w208:string)  [unwired: 14 in]
      }
      frame "Events: Register" {
        # "Do not put any code in this frame.\n(It is a separator no-op. You can make a copy of this frame to create a new UI frame)"
        n111 = call <vilib>:"Add State(s) to Queue__JKI_lib_State_Machine.vi"("State(s) in (\"\")"=w213) -> ("States Out"=w212:string)  [unwired: 14 in]
      }
      frame "Events: Unregister" {
        # "Do not put any code in this frame.\n(It is a separator no-op. You can make a copy of this frame to create a new UI frame)"
        n112 = Unregister For Events(event registration refnum=w216, error in=w215) -> (error out=w214:errorcluster)
        n113 = call <vilib>:"Add State(s) to Queue__JKI_lib_State_Machine.vi"("State(s) in (\"\")"=w219) -> ("States Out"=w218:string)  [unwired: 14 in]
      }
      frame "---------- UI ----------" {
        # "Do not put any code in this frame.\n(It is a separator no-op. You can make a copy of this frame to create a new UI frame)"
        n114 = call <vilib>:"Add State(s) to Queue__JKI_lib_State_Machine.vi"("State(s) in (\"\")"=w223) -> ("States Out"=w222:string)  [unwired: 14 in]
      }
      frame "UI: Initialize" {
        # "Initialize the User Interface, here.\n(this is called automatically, by the Macro: Init)"
        n115 = invoke class="VI" method="Default Vals.Reinit All"(error in=w236) -> (error out=w235:errorcluster)  [unwired: 2 in, 2 out]
        n116 = Current VI's Path() -> (path=w241:path)
        n117 = call "FEV_Strip & Build Path.vi"("Strip Levels"=2, "error in (no error)"=w235, "Build Path"="Data\\Models", "Path In"=w241) -> ("error out"=w239:errorcluster, "New Path Out"=w233:path)  [unwired: 5 in, 1 out]
        n118 = List Folder(path=w233) -> (folder names=w232:string[])  [unwired: 3 in, 3 out]
        n119 = Bundle By Name(cluster=w238, "File paths.Base file path"=w233, "DATA WRITE COUNT"=0, "MESSAGES"="READING THE BATTERY EMULATOR DATA") -> (w237:T4)
        n120 = property on="MODEL SELECTION" class="CmbBox"("Strings[]"=w232) -> (error out=w227:errorcluster)  [unwired: 2 in, 1 out]
        n121 = property on="CONTROL SELECTION" class="CmbBox"("Strings[]"=string[] ["CV", "CI", "CP"]) -> ()  [unwired: 2 in, 2 out]
        n122 = property on="HVHC SELECTION" class="CmbBox"("Strings[]"=string[] ["HIGH CURRENT", "HIGH VOLTAGE"]) -> ()  [unwired: 2 in, 2 out]
        n123 = call "FGV MODEL.vi"("STATES"=MODEL_CONTROL."READ") -> ("MODEL OUT"=w228:string)  [unwired: 10 in]
        n124 = call <vilib>:"Add State(s) to Queue__JKI_lib_State_Machine.vi"("State(s) in (\"\")"=w226) -> ("States Out"=w243:string)  [unwired: 14 in]
        n125 = property on="MODEL SELECTION" class="CmbBox"(error in=w227, "Value"=w228) -> ()  [unwired: 1 in, 2 out]
        "Headline" <- "Battery Emulator Auto Screen" ("Headline")
      }
      frame "UI: Cursor Set" {
        # "Argument"
        # "Set and Unset Cursor Busy.\n(Usage: \"UI: Cursor Set >> Busy|Idle\")"
        n126 = case shown="\"Idle\", Default" w244 {
          tunnel: w246 -> [w251 w253]
          tunnel: [w250 w252] -> w245
          frame "Idle", Default {
            n127 = call <vilib>:"Unset Busy.vi"("error in (no error)"=w251) -> ("error out"=w250:errorcluster)  [unwired: 10 in]
          }
          frame "Busy" {
            n128 = call <vilib>:"Set Busy.vi"("error in (no error)"=w253) -> ("error out"=w252:errorcluster)  [unwired: 9 in, 1 out]
          }
        }
        n129 = call <vilib>:"Add State(s) to Queue__JKI_lib_State_Machine.vi"("State(s) in (\"\")"=w249) -> ("States Out"=w248:string)  [unwired: 14 in]
      }
      frame "UI: Front Panel State" {
        # "Argument"
        # "Set Front Panel Open or Closed\n(Usage: \"UI: Front Panel State >> Open|Close\")"
        n130 = Unbundle By Name(w257) -> ("Core.Current VI Reference"=w256:refnum<vi>)
        n131 = case shown="\"Open\", \"Standard\", Default" w255 {
          tunnel: w259 -> [w267 w282 w293 w306 w319]
          tunnel: [w269 w283 w295 w308 w321] -> w258
          tunnel: w256 -> [w268 w280 w294 w307 w320]
          frame "Open", "Standard", Default {
            w262 = T1."Standard" ("State")
            n132 = property class="VI"(reference=w268, error in=w267) -> (reference out=w265:refnum<vi>, error out=w266:errorcluster, "FP.State"=w264:T1)
            n133 = Not Equal?(x=w264, y=w262) -> (x != y?=w263:bool)
            n134 = case shown="True" w263 {
              tunnel: [w273 w275] -> w269
              tunnel: w266 -> [w272 w275]
              tunnel: w265 -> [w271 _]
              tunnel: w262 -> [w270 _]
              frame True {
                n135 = invoke class="VI" method="FP.Open"(reference=w271, error in=w272, "Activate"=TRUE, "State"=w270) -> (error out=w273:errorcluster)  [unwired: 1 in, 4 out]
              }
              frame False {
              }
            }
          }
          frame "Close", "Closed" {
            n136 = property class="VI"(reference=w280, error in=w282) -> (reference out=w279:refnum<vi>, error out=w281:errorcluster, "FP.State"=w277:T1)
            n137 = Not Equal?(x=w277, y=T1."Closed" ("Front Panel Window:State")) -> (x != y?=w276:bool)
            n138 = case shown="True" w276 {
              tunnel: [w284 w287] -> w283
              tunnel: w281 -> [w284 w286]
              tunnel: w279 -> [_ w285]
              frame False {
              }
              frame True {
                n139 = invoke class="VI" method="FP.Close"(reference=w285, error in=w286) -> (error out=w287:errorcluster)  [unwired: 1 in, 2 out]
              }
            }
          }
          frame "Hidden", "Hide" {
            w288 = T1."Hidden" ("State")
            n140 = property class="VI"(reference=w294, error in=w293) -> (reference out=w291:refnum<vi>, error out=w292:errorcluster, "FP.State"=w290:T1)
            n141 = Not Equal?(x=w290, y=w288) -> (x != y?=w289:bool)
            n142 = case shown="True" w289 {
              tunnel: [w299 w300] -> w295
              tunnel: w292 -> [w298 w300]
              tunnel: w291 -> [w297 _]
              tunnel: w288 -> [w296 _]
              frame True {
                n143 = invoke class="VI" method="FP.Open"(reference=w297, error in=w298, "State"=w296) -> (error out=w299:errorcluster)  [unwired: 2 in, 4 out]
              }
              frame False {
              }
            }
          }
          frame "Minimize", "Minimized" {
            w301 = T1."Minimized" ("State")
            n144 = property class="VI"(reference=w307, error in=w306) -> (reference out=w304:refnum<vi>, error out=w305:errorcluster, "FP.State"=w303:T1)
            n145 = Not Equal?(x=w303, y=w301) -> (x != y?=w302:bool)
            n146 = case shown="True" w302 {
              tunnel: [w312 w313] -> w308
              tunnel: w305 -> [w311 w313]
              tunnel: w304 -> [w310 _]
              tunnel: w301 -> [w309 _]
              frame True {
                n147 = invoke class="VI" method="FP.Open"(reference=w310, error in=w311, "State"=w309) -> (error out=w312:errorcluster)  [unwired: 2 in, 4 out]
              }
              frame False {
              }
            }
          }
          frame "Maximize", "Maximized" {
            w314 = T1."Maximized" ("State")
            n148 = property class="VI"(reference=w320, error in=w319) -> (reference out=w317:refnum<vi>, error out=w318:errorcluster, "FP.State"=w316:T1)
            n149 = Not Equal?(x=w316, y=w314) -> (x != y?=w315:bool)
            n150 = case shown="True" w315 {
              tunnel: [w325 w326] -> w321
              tunnel: w318 -> [w324 w326]
              tunnel: w317 -> [w323 _]
              tunnel: w314 -> [w322 _]
              frame True {
                n151 = invoke class="VI" method="FP.Open"(reference=w323, error in=w324, "State"=w322) -> (error out=w325:errorcluster)  [unwired: 2 in, 4 out]
              }
              frame False {
              }
            }
          }
        }
        n152 = call <vilib>:"Add State(s) to Queue__JKI_lib_State_Machine.vi"("State(s) in (\"\")"=w261, "State(s) at Back (\"\")"="DATABASE: READ DATABASE" ("State(s) at Back (\"\")")) -> ("States Out"=w260:string)  [unwired: 13 in]
      }
      frame "---------- Macro ----------" {
        # "Do not put any code in this frame.\n(It is a separator no-op. You can make a copy of this frame to create a new Macro frame)"
        n153 = call <vilib>:"Add State(s) to Queue__JKI_lib_State_Machine.vi"("State(s) in (\"\")"=w330) -> ("States Out"=w329:string)  [unwired: 14 in]
      }
      frame "Macro: Initialize" {
        # "Initialization Macro\n(This is called once, when the VI starts)"
        n154 = call <vilib>:"Add State(s) to Queue__JKI_lib_State_Machine.vi"("State(s) in Front (\"\")"="Data: Initialize\nInitialize Core Data\nEvents: Register\nUI: Initialize\nUI: Front Panel State >> Open", "State(s) in (\"\")"=w335) -> ("States Out"=w334:string)  [unwired: 13 in]
      }
      frame "Macro: Exit" {
        # "Exit Macro\n(This is called once, when the VI exits)"
        n155 = Unbundle By Name(w340) -> ("Core.Close Panel on Exit?"=w350:bool, "CHANGE REQ?"=w337:bool)
        n156 = case shown="True" w337 {
          tunnel: w345 -> [w355 w361]
          tunnel: [w354 w361] -> w344
          tunnel: [w353 TRUE ("T button?")] -> w338
          frame False {
            n157 = flat-sequence {
              tunnel: w355 -> [w359]
              tunnel: [w359] -> w354
              tunnel: [w356] -> w353
              frame #0 {
                n158 = Two Button Dialog(message="Do you want to change the data on battery emulator??", 1:"NO" ("F button name (\"Cancel\")"), 2:"YES" ("T button name (\"OK\")")) -> (T button?=w356:bool)
              }
            }
          }
          frame True {
          }
        }
        n159 = Select(t="UI: Front Panel State >> Close", s=w350, f="") -> (s? t:f=w347:string)
        n160 = call <vilib>:"Add State(s) to Queue__JKI_lib_State_Machine.vi"("State(s) in (\"\")"=w347, "State(s) at Back (\"\")"="Data: Cleanup\nEvents: Unregister\nExit") -> ("States Out"=w343:string)  [unwired: 13 in]
        n161 = Select(t="", s=w338, f=w343) -> (s? t:f=w341:string)
        n162 = call <vilib>:"Add State(s) to Queue__JKI_lib_State_Machine.vi"("State(s) in Front (\"\")"=w341, "State(s) in (\"\")"=w352) -> ("States Out"=w351:string)  [unwired: 13 in]
        n163 = Bundle By Name(cluster=w340, "CHANGE REQ?"=w338, "DATA WRITE COUNT"=0) -> (w339:T4)
      }
      frame "---------- DATABSE ----------" {
        # "Template Separator\n(You can make a copy of, or modify, this frame)"
        n164 = call <vilib>:"Add State(s) to Queue__JKI_lib_State_Machine.vi"("State(s) in (\"\")"=w366) -> ("States Out"=w365:string)  [unwired: 14 in]
      }
      frame "DATABASE: READ DATABASE" {
        # "Your code here.\n(You can make a copy of, or modify, this frame)"
        n165 = Unbundle By Name(w370) -> ("BATTERY EMULATOR"=w384:T5, "File paths.Model File path"=w386:path)
        n166 = Build Path(base path=w386, name or relative path="Battery Emulator.txt") -> (appended path=w387:path)
        n167 = Read from Binary File(5:w384, 8:w389, 11:w387) -> (0:w385:errorcluster, 2:w368:T5)  [unwired: 3 in, 2 out]
        n168 = Cluster To Array(cluster=w368) -> (array=w383:string[])
        n169 = Index Array(array=w383) -> (element #1=w382:string, element #2=w381:string, element #3=w380:string, element #4=w379:string, element #5=w378:string, element #6=w377:string, element #7=w376:string, element #8=w375:string, element #9=w374:string, element #10=w373:string, element #11=w372:string)  [unwired: 11 in]
        n170 = property on="HVHC SELECTION" class="CmbBox"("Value"=w382) -> ()  [unwired: 2 in, 2 out]
        n171 = property on="CONTROL SELECTION" class="CmbBox"("Value"=w381) -> ()  [unwired: 2 in, 2 out]
        n172 = property on="CV VOLTAGE" class="Str"("Value"=w380) -> ()  [unwired: 2 in, 2 out]
        n173 = property on="CV CURRENT" class="Str"("Value"=w379) -> ()  [unwired: 2 in, 2 out]
        n174 = property on="CV POWER" class="Str"("Value"=w378) -> ()  [unwired: 2 in, 2 out]
        n175 = property on="CI VOLTAGE" class="Str"("Value"=w377) -> ()  [unwired: 2 in, 2 out]
        n176 = property on="CI CURRENT" class="Str"("Value"=w376) -> ()  [unwired: 2 in, 2 out]
        n177 = property on="CI POWER" class="Str"("Value"=w375) -> ()  [unwired: 2 in, 2 out]
        n178 = property on="CP CURRENT" class="Str"("Value"=w373) -> ()  [unwired: 2 in, 2 out]
        n179 = property on="CP VOLTAGE" class="Str"("Value"=w374) -> ()  [unwired: 2 in, 2 out]
        n180 = property on="CP POWER" class="Str"("Value"=w372) -> ()  [unwired: 2 in, 2 out]
        n181 = call <vilib>:"Add State(s) to Queue__JKI_lib_State_Machine.vi"("State(s) in (\"\")"=w391, "State(s) at Back (\"\")"="DATABASE: WRITE DATA" ("State(s) at Back (\"\")")) -> ("States Out"=w390:string)  [unwired: 13 in]
        n182 = Bundle By Name(cluster=w370, "BATTERY EMULATOR"=w368, "MESSAGES"="DATA IS WRITING TO BATTERY EMULATOR") -> (w369:T4)
      }
      frame "DATABASE: READ BATTERY DATA" {
        # "Your code here.\n(You can make a copy of, or modify, this frame)"
        n183 = call "Stall Data Flow.vim"("value in"=w410, "milliseconds to wait"=u32 15000) -> ("value out"=w409:errorcluster)  [unwired: 1 out]
        n184 = call-poly <vilib>:"XNET Create Session.vi"("signal list"=refnum<k21>[] ["OutputCurrent\nFEV_150KW-R0", "OutputPower\nFEV_150KW-R0", "OutputVoltage\nFEV_150KW-R0", "ErrorControlSelErr\nFEV_150KW-R0", "ErrorNotInRemoteMode\nFEV_150KW-R0", "ErrorPowerSetOutofRange\nFEV_150KW-R0", "ErrorVoltSetOutofRange\nFEV_150KW-R0", "ErrorWrongHVSel\nFEV_150KW-R0", "PowerSwitchONStatus\nFEV_150KW-R0", "StatusDcpsFault\nFEV_150KW-R0", "StatusHCHV_selection\nFEV_150KW-R0", "HandShakeAcknowledge\nFEV_150KW-R0", "RemoteDisplaySelAck\nFEV_150KW-R0", "Select_CVCICPAck\nFEV_150KW-R0", "Select_HVHC_Ack\nFEV_150KW-R0", "CV_SetCurrentLimitAck\nFEV_150KW-R0", "CV_SetPowerLimitAck\nFEV_150KW-R0", "CV_SetVoltageAck\nFEV_150KW-R0", "UpdateCmdAcknowledge\nFEV_150KW-R0"] ("Sigs 2"), "interface"=refnum<k21> "CAN2" ("Select Interface"), "error in (no error)"=w409) -> ("session out"=w433:refnum<k21>, "error out"=w434:errorcluster)  [unwired: 1 in, 10 out]
        n185 = Unbundle By Name(w402) -> ("BATTERY EMULATOR"=w407:T5, "DATA WRITE COUNT"=w400:i32)
        n186 = call <vilib>:"XNET Start.vi"("session in"=w433, "error in (no error)"=w434) -> ("session out"=w435:refnum<k21>, "error out"=w436:errorcluster)  [unwired: 12 in]
        n187 = call "Stall Data Flow.vim"("value in"=w436, "milliseconds to wait"=u32 1000) -> ("value out"=w432:errorcluster)  [unwired: 1 out]
        n188 = call-poly <vilib>:"XNET Read.vi"("session in"=w435, "error in (no error)"=w432) -> ("data"=w406:dbl[], "error out"=w428:errorcluster)  [unwired: 11 in, 1 out]
        n189 = Number To Fractional String(number=w406) -> (F-format string=w425:string[])  [unwired: 3 in]
        n190 = Index Array(array=w425, index #1=13 ("index"), index #2=10 ("index")) -> (element #1=w426:string, element #2=w419:string)  [unwired: 1 in, 1 out]
        n191 = Index Array(array=w425) -> (element #1=w424:string, element #2=w423:string, element #3=w422:string)  [unwired: 3 in]
        n192 = Equal?(x=w419, y="224") -> (x = y?=w417:bool)
        n193 = case shown="\"226\", Default" w426 {
          tunnel: w424 -> [w445 w452 w459]
          tunnel: w423 -> [w444 w451 w458]
          tunnel: w422 -> [w443 w450 w457]
          tunnel: ["CV" "CI" "CP"] -> w420
          tunnel: [TRUE FALSE FALSE] -> w413
          tunnel: [FALSE FALSE TRUE] -> w412
          tunnel: [FALSE TRUE FALSE] -> w411
          frame "226", Default {
            "CV POWER" <- w443
            "CV VOLTAGE" <- w445
            "CV CURRENT" <- w444
          }
          frame "227" {
            "CI VOLTAGE" <- w452
            "CI CURRENT" <- w451
            "CI POWER" <- w450
          }
          frame "228" {
            "CP POWER" <- w457
            "CP CURRENT" <- w458
            "CP VOLTAGE" <- w459
          }
        }
        "CONTROL SELECTION" <- w420
        n194 = Select(t="HIGH CURRENT", s=w417, f="HIGH VOLTAGE") -> (s? t:f=→"HVHC SELECTION":string)
        n195 = Increment(x=w400) -> (x+1=w398:i32)
        n196 = property on="CI VOLTAGE" class="Str"("Visible"=w411) -> ()  [unwired: 2 in, 2 out]
        n197 = property on="CP VOLTAGE" class="Str"("Visible"=w412) -> ()  [unwired: 2 in, 2 out]
        n198 = property on="CP POWER" class="Str"("Visible"=w412) -> ()  [unwired: 2 in, 2 out]
        n199 = property on="CI CURRENT" class="Str"("Visible"=w411) -> ()  [unwired: 2 in, 2 out]
        n200 = property on="CP CURRENT" class="Str"("Visible"=w412) -> ()  [unwired: 2 in, 2 out]
        n201 = property on="CI POWER" class="Str"("Visible"=w411) -> ()  [unwired: 2 in, 2 out]
        n202 = property on="CV VOLTAGE" class="Str"("Visible"=w413) -> ()  [unwired: 2 in, 2 out]
        n203 = property on="CV CURRENT" class="Str"("Visible"=w413) -> ()  [unwired: 2 in, 2 out]
        n204 = property on="CV POWER" class="Str"("Visible"=w413) -> ()  [unwired: 2 in, 2 out]
        n205 = call "CHECK BATT DATA.vi"("DATA"=w406, "BATTERY EMULATOR"=w407) -> ("result"=w395:bool)  [unwired: 9 in]
        n206 = Select(t="BATTERY EMULATOR IS READY", s=w395, f="WRITING DATA AGAIN!! DATA WRITE IS NOT MATCHED WITH CURRENT DATA") -> (s? t:f=w392:string)
        n207 = Bundle By Name(cluster=w402, "MESSAGES"=w392, "DATA WRITE COUNT"=w398) -> (w401:T4)
        n208 = Greater Or Equal?(x=w398, y=2.0) -> (x >= y?=w397:bool)
        n209 = Or(x=w395, y=w397) -> (x .or. y?=w396:bool)
        n210 = Select(t="Data: Cleanup\nEvents: Unregister\nExit" ("State(s) at Back (\"\")"), s=w396, f="DATABASE: WRITE DATA" ("State(s) at Back (\"\")")) -> (s? t:f=w403:string)
        n211 = call <vilib>:"Add State(s) to Queue__JKI_lib_State_Machine.vi"("State(s) in (\"\")"=w438, "State(s) at Back (\"\")"=w403) -> ("States Out"=w437:string)  [unwired: 13 in]
      }
      frame "DATABASE: WRITE DATA" {
        w485 = refnum<k21>[] ["HandShakeCmd\nFEV_150KW-R0", "RemoteDisplaySel\nFEV_150KW-R0", "Select_CVCICP\nFEV_150KW-R0", "Select_HVHC\nFEV_150KW-R0", "CV_SetCurrentLimit\nFEV_150KW-R0", "CV_SetPowerLimit\nFEV_150KW-R0", "CV_SetVoltage\nFEV_150KW-R0", "B_RemoteToDcps.Reserved\nFEV_150KW-R0", "CI_SetCurrent\nFEV_150KW-R0", "CI_SetPowerLimit\nFEV_150KW-R0", "CI_SetVoltageLimit\nFEV_150KW-R0", "C_RemoteToDcps.Reserved\nFEV_150KW-R0", "CP_SetCurrentLimit\nFEV_150KW-R0", "CP_SetPower\nFEV_150KW-R0", "CP_SetVoltageLimit\nFEV_150KW-R0", "D_RemoteToDcps.UpdateCmd\nFEV_150KW-R0", "HandShakeAcknowledge\nFEV_150KW-R0", "RemoteDisplaySelAck\nFEV_150KW-R0", "Select_CVCICPAck\nFEV_150KW-R0", "Select_HVHC_Ack\nFEV_150KW-R0", "CV_SetCurrentLimitAck\nFEV_150KW-R0", "CV_SetPowerLimitAck\nFEV_150KW-R0", "CV_SetVoltageAck\nFEV_150KW-R0", "PowerSwitchONStatus\nFEV_150KW-R0", "CI_SetCurrentAck\nFEV_150KW-R0", "CI_SetPowerLimitAck\nFEV_150KW-R0", "CI_SetVoltageLimitAck\nFEV_150KW-R0", "ErrorControlSelErr\nFEV_150KW-R0", "ErrorCurSetOutofRange\nFEV_150KW-R0", "ErrorNotInRemoteMode\nFEV_150KW-R0", "ErrorPowerSetOutofRange\nFEV_150KW-R0", "ErrorVoltSetOutofRange\nFEV_150KW-R0", "ErrorWrongHVSel\nFEV_150KW-R0", "Reserved_Status\nFEV_150KW-R0", "CP_SetCurrentLimitAck\nFEV_150KW-R0", "CP_SetPowerAck\nFEV_150KW-R0", "CP_SetVoltageLimitAck\nFEV_150KW-R0", "UpdateCmdAcknowledge\nFEV_150KW-R0", "OutputCurrent\nFEV_150KW-R0", "OutputPower\nFEV_150KW-R0", "OutputVoltage\nFEV_150KW-R0", "StatusDcpsFault\nFEV_150KW-R0", "StatusDcpsON\nFEV_150KW-R0", "StatusDcpsOverload\nFEV_150KW-R0", "StatusDcpsTrip\nFEV_150KW-R0", "StatusHCHV_selection\nFEV_150KW-R0", "StatusInputOverVolt\nFEV_150KW-R0", "StatusInputUnderVolt\nFEV_150KW-R0", "StatusMainsHealthy\nFEV_150KW-R0", "StatusOutputOverVolt\nFEV_150KW-R0", "StatusOutputUnderVolt\nFEV_150KW-R0", "StatusOverTemperature\nFEV_150KW-R0", "StatusRemoteLocal\nFEV_150KW-R0"] ("Sigs")
        w487 = refnum<k21> "CAN2" ("Select Interface")
        # "Your code here.\n(You can make a copy of, or modify, this frame)"
        n212 = Unbundle By Name(w476) -> ("BATTERY EMULATOR"=w471:T5)
        n213 = Delete From Array(array=refnum<k21>[] ["HandShakeCmd\nFEV_150KW-R0", "RemoteDisplaySel\nFEV_150KW-R0", "Select_HVHC", "Select_CVCICP", "CV_SetCurrentLimit\nFEV_150KW-R0", "CV_SetPowerLimit\nFEV_150KW-R0", "CV_SetVoltage\nFEV_150KW-R0", "B_RemoteToDcps.Reserved\nFEV_150KW-R0", "CI_SetCurrent\nFEV_150KW-R0", "CI_SetPowerLimit\nFEV_150KW-R0", "CI_SetVoltageLimit\nFEV_150KW-R0", "C_RemoteToDcps.Reserved\nFEV_150KW-R0", "CP_SetCurrentLimit\nFEV_150KW-R0", "CP_SetPower\nFEV_150KW-R0", "CP_SetVoltageLimit\nFEV_150KW-R0", "D_RemoteToDcps.UpdateCmd\nFEV_150KW-R0", "HandShakeAcknowledge\nFEV_150KW-R0", "RemoteDisplaySelAck\nFEV_150KW-R0", "Select_CVCICPAck\nFEV_150KW-R0", "Select_HVHC_Ack\nFEV_150KW-R0", "CV_SetCurrentLimitAck\nFEV_150KW-R0", "CV_SetPowerLimitAck\nFEV_150KW-R0", "CV_SetVoltageAck\nFEV_150KW-R0", "PowerSwitchONStatus\nFEV_150KW-R0", "CI_SetCurrentAck\nFEV_150KW-R0", "CI_SetPowerLimitAck\nFEV_150KW-R0", "CI_SetVoltageLimitAck\nFEV_150KW-R0", "ErrorControlSelErr\nFEV_150KW-R0", "ErrorCurSetOutofRange\nFEV_150KW-R0", "ErrorNotInRemoteMode\nFEV_150KW-R0", "ErrorPowerSetOutofRange\nFEV_150KW-R0", "ErrorVoltSetOutofRange\nFEV_150KW-R0", "ErrorWrongHVSel\nFEV_150KW-R0", "Reserved_Status\nFEV_150KW-R0", "CP_SetCurrentLimitAck\nFEV_150KW-R0", "CP_SetPowerAck\nFEV_150KW-R0", "CP_SetVoltageLimitAck\nFEV_150KW-R0", "UpdateCmdAcknowledge\nFEV_150KW-R0", "OutputCurrent\nFEV_150KW-R0", "OutputPower\nFEV_150KW-R0", "OutputVoltage\nFEV_150KW-R0", "StatusDcpsFault\nFEV_150KW-R0", "StatusDcpsON\nFEV_150KW-R0", "StatusDcpsOverload\nFEV_150KW-R0", "StatusDcpsTrip\nFEV_150KW-R0", "StatusHCHV_selection\nFEV_150KW-R0", "StatusInputOverVolt\nFEV_150KW-R0", "StatusInputUnderVolt\nFEV_150KW-R0", "StatusMainsHealthy\nFEV_150KW-R0", "StatusOutputOverVolt\nFEV_150KW-R0", "StatusOutputUnderVolt\nFEV_150KW-R0", "StatusOverTemperature\nFEV_150KW-R0", "StatusRemoteLocal\nFEV_150KW-R0"] ("Sigs 3"), length=4, index=0) -> (deleted portion=w496:refnum<k21>[])  [unwired: 1 out]
        n214 = call "BATT DATA.vi"("BATTERY EMULATOR"=w471) -> ("MODEL SELECTION"=w470:dbl, "CONTROL SELECTION"=w469:dbl, "VOLTAGE"=w463:dbl, "CURRENT"=w462:dbl, "POWER"=w461:dbl)  [unwired: 14 in]
        n215 = Replace Array Subset(array=dbl[] [238.0, 235.0, 224.0, 226.0] ("data 3"), new element #1=w470, index #1=2 ("index"), new element #2=w469, index #2=3 ("index")) -> (w472:dbl[])
        n216 = call-poly <vilib>:"XNET Create Session.vi"("signal list"=w496, "interface"=w487, "error in (no error)"=w478) -> ("session out"=w491:refnum<k21>, "error out"=w492:errorcluster)  [unwired: 11 out]
        n217 = Index Array(array=w485, index=15 ("Index")) -> (element=w490:refnum<k21>)
        n218 = call-poly <vilib>:"XNET Write.vi"("session in"=w491, "data"=w472, "error in (no error)"=w492) -> ("error out"=w495:errorcluster)  [unwired: 11 in, 1 out]
        n219 = Delete From Array(array=w485, length=3, index=4) -> (deleted portion=w499:refnum<k21>[])  [unwired: 1 out]
        n220 = Build Array(w490) -> (w503:refnum<k21>[])
        n221 = call "Stall Data Flow.vim"("value in"=w495, "milliseconds to wait"=u32 1000) -> ("value out"=w498:errorcluster)  [unwired: 1 out]
        n222 = Build Array (concatenate)(w499, w503) -> (w500:refnum<k21>[])
        n223 = call-poly <vilib>:"XNET Create Session.vi"("signal list"=w500, "interface"=w487, "error in (no error)"=w498) -> ("session out"=w494:refnum<k21>, "error out"=w493:errorcluster)  [unwired: 11 out]
        n224 = Replace Array Subset(array=dbl[] [0.0, 0.0, 0.0, 161.0] ("data"), new element #1=w463, index #1=0 ("index"), new element #2=w462, index #2=1 ("index"), new element #3=w461, index #3=2 ("index")) -> (w465:dbl[])
        n225 = call-poly <vilib>:"XNET Write.vi"("session in"=w494, "data"=w465, "error in (no error)"=w493) -> ("error out"=w497:errorcluster)  [unwired: 11 in, 1 out]
        n226 = call <vilib>:"Add State(s) to Queue__JKI_lib_State_Machine.vi"("State(s) in (\"\")"=w506, "State(s) at Back (\"\")"="DATABASE: READ BATTERY DATA" ("State(s) at Back (\"\")")) -> ("States Out"=w505:string)  [unwired: 13 in]
        n227 = call "Stall Data Flow.vim"("value in"=w497, "milliseconds to wait"=u32 10000) -> ("value out"=w504:errorcluster)  [unwired: 1 out]
        n228 = call-poly <vilib>:"XNET Create Session.vi"("signal list"=w503, "interface"=w487, "error in (no error)"=w504) -> ("session out"=w501:refnum<k21>, "error out"=w502:errorcluster)  [unwired: 11 out]
        n229 = call-poly <vilib>:"XNET Write.vi"("session in"=w501, "data"=dbl[] [160.0], "error in (no error)"=w502) -> ("error out"=w477:errorcluster)  [unwired: 11 in, 1 out]
      }
    }
    n230 = Unbundle By Name(w15) -> ("MESSAGES"=→"MESSAGES":string)
  }
  "error out" <- w1
